vi "VariableScan_StandAlone.vi"() -> ()   [LabVIEW 2018]
uses:
  VariableScan_Cluster.ctl
panel:
  in  "Abort":bool
  in  "Text File Path":path=path "C:/CuspControl/GPIB and Network/VariableScan.txt"
  in  "stop":bool
  in  "Variable Cluster":T1={"Values"=[1.0, 2.0], "Action"=0, "Inst."=0, "# Elements"=2, "Next Element"=0, "First Val"=1.0, "Final Val"=2.0, "Update Array"=FALSE, "Description"="", "Variable Type"=0, "Scan Now"=FALSE, "# Act/Inst."=2, "Electrodes_range"=[], "Parameter Name"="RW&f_start (Hz)", "# Passes"=1} {"Variable Type" items=["Duration (s)", "Voltage (V)", "Parameter", "Repetitions"]; "Final Val" format="%_6p"; "First Val" format="%_6p"; "Values" format="%_6p"}
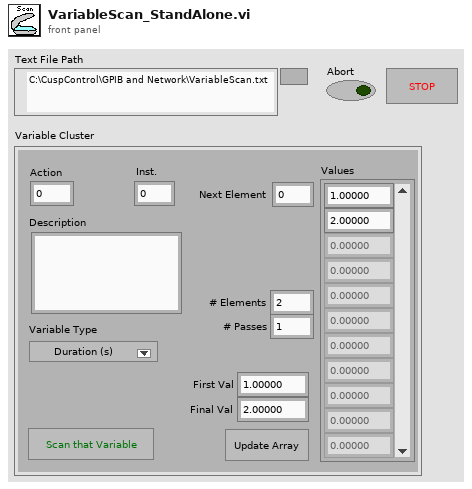
[diagram p1: front panel]
types:
  T1 = typedef "VariableScan_Cluster.ctl" = cluster{"Values":dbl[], "Action":i32, "Inst.":i32, "# Elements":i32, "Next Element":i32, "First Val":dbl, "Final Val":dbl, "Update Array":bool, "Description":string, "Variable Type":u16, "Scan Now":bool, "# Act/Inst.":i32, "Electrodes_range":i32[], "Parameter Name":string, "# Passes":i32}
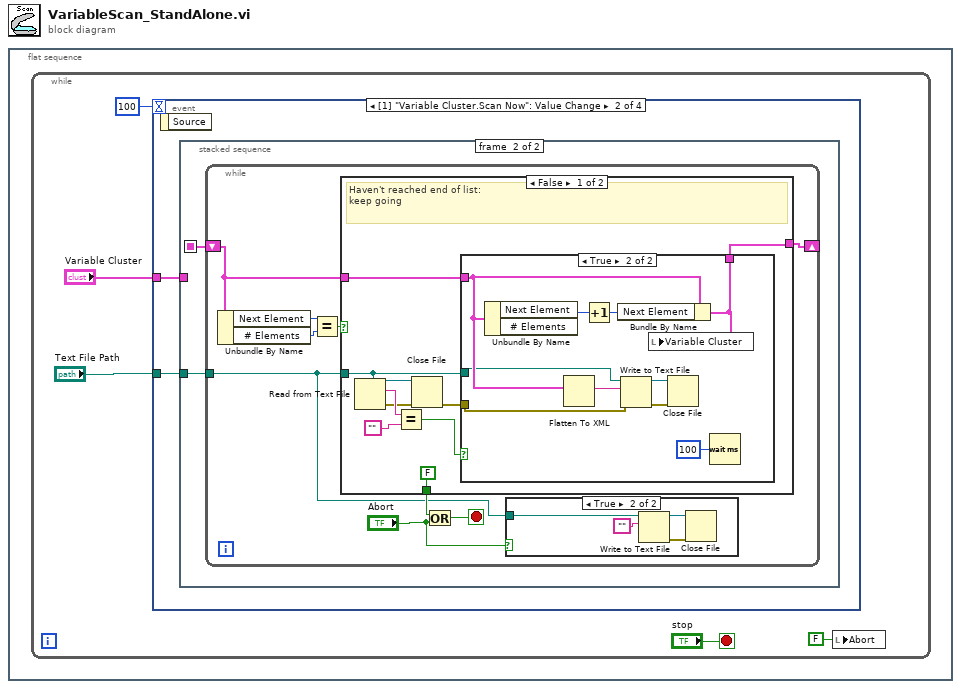
[diagram p0: block diagram]
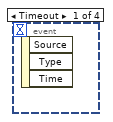
[diagram p2: hidden frame]
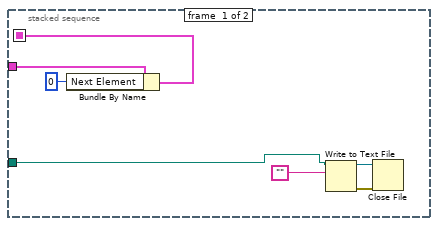
[diagram p3: hidden frame]
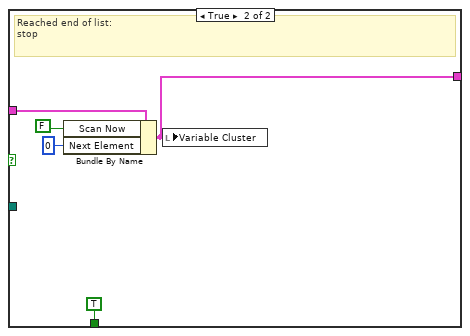
[diagram p6: hidden frame]
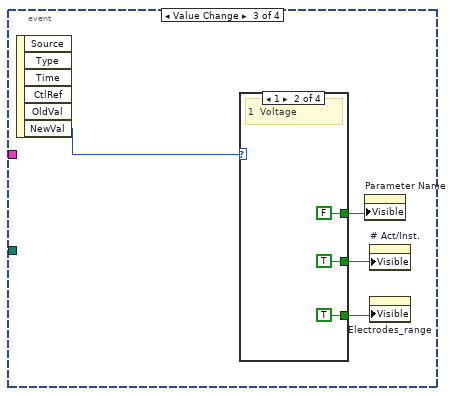
[diagram p7: hidden frame]
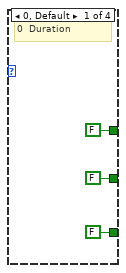
[diagram p8: hidden frame]
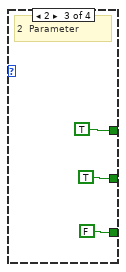
[diagram p9: hidden frame]
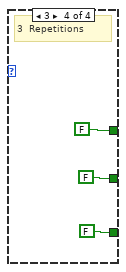
[diagram p10: hidden frame]
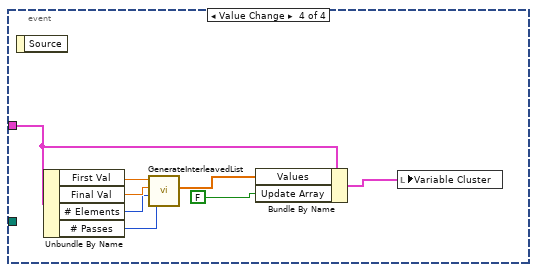
[diagram p11: hidden frame]
diagram:
  n1 = flat-sequence {
    frame #0 {
      n2 = while {
        stop <- "stop" stop-if-true
        n3 = event shown="[1] \"Variable Cluster.Scan Now\": Value Change" {
          selector: _ -> [_ _ _ _]
          dyn-events: _ -> [_ _ _ _]
          timeout: 100 -> [_ _ _ _]
          tunnel: "Variable Cluster" -> [_ w7 _ w73]
          tunnel: "Text File Path" -> [_ w6 _ _]
          event Timeout {
            n4 = event-data() -> ()  [unwired: 1 in, 3 out]
          }
          event Value Change {
            n5 = event-data() -> ()  [unwired: 1 in, 1 out]
            n6 = stacked-sequence {
              seq-local: [w9 _] -> [_ w15]
              tunnel: w7 -> [w14 _]
              tunnel: w6 -> [w10 w16]
              frame #0 {
                n7 = Bundle By Name(cluster=w14, "Next Element"=0) -> (w9:T1)
                n8 = Write to Text File(file (use dialog)=w10, text="") -> (refnum out=w11:refnum<file>, error out=w12:errorcluster)  [unwired: 2 in, 1 out]
                n9 = Close File(refnum=w11, error in=w12) -> ()  [unwired: 2 out]
              }
              frame #1 {
                n10 = while {
                  tunnel: w16 -> [w17]
                  shift-right: [w21] -> _
                  shift-left: w15 -> [w25]
                  stop <- w19 stop-if-true
                  n11 = Unbundle By Name(w25) -> ("Next Element"=w24:i32, "# Elements"=w22:i32)
                  n12 = Equal?(x=w24, y=w22) -> (x = y?=w23:bool)
                  n13 = case shown="False" w23 {
                    tunnel: w25 -> [w39 w54]
                    tunnel: w17 -> [w38 _]
                    tunnel: [FALSE TRUE] -> w20
                    tunnel: [w33 w51] -> w21
                    frame False {
                      # "Haven't reached end of list:\nkeep going"
                      n14 = Read from Text File(file (use dialog)=w38) -> (refnum out=w32:refnum<file>, text=w35:string, error out=w31:errorcluster)  [unwired: 3 in, 1 out]
                      n15 = Equal?(x=w35, y="") -> (x = y?=w34:bool)
                      n16 = Close File(refnum=w32, error in=w31) -> (error out=w30:errorcluster)  [unwired: 1 out]
                      n17 = case shown="True" w34 {
                        tunnel: w39 -> [w40 w48]
                        tunnel: w38 -> [_ w47]
                        tunnel: [w40 w43] -> w33
                        tunnel: w30 -> [_ w42]
                        frame False {
                          # "wait for Cue to run"
                        }
                        frame True {
                          n18 = Unbundle By Name(w48) -> ("Next Element"=w49:i32)  [unwired: 1 out]
                          n19 = Flatten To XML(anything=w48) -> (xml string=w44:string)
                          n20 = Increment(x=w49) -> (x+1=w50:i32)
                          n21 = Bundle By Name(cluster=w48, "Next Element"=w50) -> (w43:T1)
                          n22 = Write to Text File(file (use dialog)=w47, text=w44, error in=w42) -> (refnum out=w45:refnum<file>, error out=w46:errorcluster)  [unwired: 1 in, 1 out]
                          n23 = local write "Variable Cluster"(w43) -> ()
                          n24 = Close File(refnum=w45, error in=w46) -> ()  [unwired: 2 out]
                          n25 = Wait (ms)(milliseconds to wait=u32 100) -> ()  [unwired: 1 out]
                        }
                      }
                    }
                    frame True {
                      # "Reached end of list:\nstop"
                      n26 = Bundle By Name(cluster=w54, "Scan Now"=FALSE ("Value (Signaling)"), "Next Element"=0) -> (w51:T1)
                      n27 = local write "Variable Cluster"(w51) -> ()
                    }
                  }
                  n28 = Or(x=w20, y="Abort") -> (x .or. y?=w19:bool)
                  n29 = case shown="True" "Abort" {
                    tunnel: w17 -> [_ w26]
                    frame False {
                    }
                    frame True {
                      n30 = Write to Text File(file (use dialog)=w26, text="") -> (refnum out=w29:refnum<file>, error out=w28:errorcluster)  [unwired: 2 in, 1 out]
                      n31 = Close File(refnum=w29, error in=w28) -> ()  [unwired: 2 out]
                    }
                  }
                }
              }
            }
          }
          event Value Change {
            n32 = event-data() -> ("NewVal"=w56:u16)  [unwired: 1 in, 5 out]
            n33 = case shown="1" w56 {
              tunnel: [FALSE ("Visible") TRUE ("Visible") FALSE ("Visible") FALSE ("Visible")] -> w59
              tunnel: [FALSE ("Visible") TRUE ("Visible") TRUE ("Visible") FALSE ("Visible")] -> w58
              tunnel: [FALSE ("Visible") FALSE ("Visible") TRUE ("Visible") FALSE ("Visible")] -> w57
              frame 0, Default {
                # "0  Duration"
              }
              frame 1 {
                # "1  Voltage"
              }
              frame 2 {
                # "2  Parameter"
              }
              frame 3 {
                # "3  Repetitions"
              }
            }
            n34 = property on="Parameter Name" class="Str"("Visible"=w57) -> ()  [unwired: 2 in, 2 out]
            n35 = property on="# Act/Inst." class="DigNum (strict)"("Visible"=w58) -> ()  [unwired: 2 in, 2 out]
            n36 = property on="Electrodes_range" class="Arr (strict)"("Visible"=w59) -> ()  [unwired: 2 in, 2 out]
          }
          event Value Change {
            n37 = event-data() -> ()  [unwired: 1 in, 1 out]
            n38 = Unbundle By Name(w73) -> ("First Val"=w78:dbl, "Final Val"=w77:dbl, "# Elements"=w76:i32, "# Passes"=w75:i32)
            n39 = call "GenerateInterleavedList.vi"("# passes"=w75, "# points"=w76, "Stop"=w77, "Start"=w78) -> ("Array"=w74:dbl[])  [unwired: 2 in, 1 out]
            n40 = Bundle By Name(cluster=w73, "Values"=w74, "Update Array"=FALSE) -> (w79:T1)
            n41 = local write "Variable Cluster"(w79) -> ()
          }
        }
        n42 = local write "Abort"(FALSE ("Abort")) -> ()
      }
    }
  }
